vi "GetStepConfig.vi"(11 "error in":errorcluster) -> (4 "Wash Array":T1[](array[typedef]), 15 "error out":errorcluster)   [LabVIEW 2016, in "CarWashTest.lvlib"]
doc: "Wash Configuration"
uses:
  CarWashTest.lvlib
  Controls/WashStepConfig.ctl
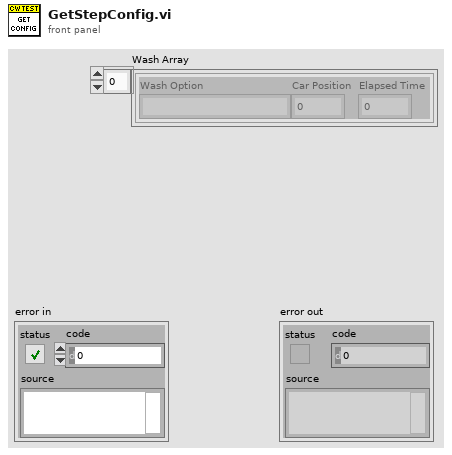
[diagram p1: front panel]
types:
  T1 = typedef "CarWashTest.lvlib/WashStepConfig.ctl" = cluster{"Wash Option":string, "Car Position":i32, "Elapsed Time":dbl}
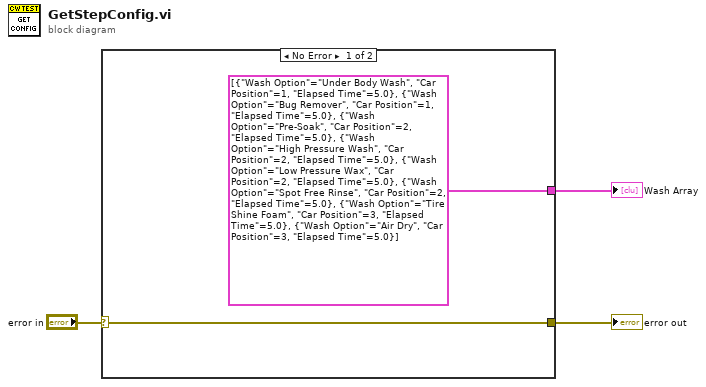
[diagram p0: block diagram]
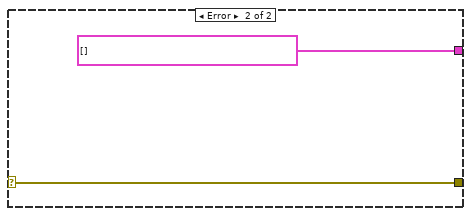
[diagram p2: hidden frame]
diagram:
  n1 = case shown="No Error" "error in" {
    selector: "error in" -> [w4 w7]
    tunnel: [T1[] [{"Wash Option"="Under Body Wash", "Car Position"=1, "Elapsed Time"=5.0}, {"Wash Option"="Bug Remover", "Car Position"=1, "Elapsed Time"=5.0}, {"Wash Option"="Pre-Soak", "Car Position"=2, "Elapsed Time"=5.0}, {"Wash Option"="High Pressure Wash", "Car Position"=2, "Elapsed Time"=5.0}, {"Wash Option"="Low Pressure Wax", "Car Position"=2, "Elapsed Time"=5.0}, {"Wash Option"="Spot Free Rinse", "Car Position"=2, "Elapsed Time"=5.0}, {"Wash Option"="Tire Shine Foam", "Car Position"=3, "Elapsed Time"=5.0}, {"Wash Option"="Air Dry", "Car Position"=3, "Elapsed Time"=5.0}] ("Wash Array") T1[] [] ("Wash Array")] -> w3
    tunnel: [w4 w7] -> w1
    frame No Error {
    }
    frame Error {
    }
  }
  "Wash Array" <- w3
  "error out" <- w1
